vi "_Write.vi"(8 "error in (no error)":errorcluster, 9 "Timeout S (0)":dbl, 10 "Data":string, 11 "DeploySerialResource in":refnum<class "SerialResource.lvclass">) -> (0 "error out":errorcluster, 2 "Bytes Written":i32, 3 "DeploySerialResource out":refnum<class "SerialResource.lvclass">)   [LabVIEW 2020, in "PicoG-Core.lvlib" / "SerialResource.lvclass"]
uses:
  SerialResource.lvclass
  <vilib>/IlluminatedG/IG Serial Stream/Stream-Serial/Serial Client/Serial Client.lvclass
  <vilib>/IlluminatedG/lv-stream/stream/Stream.lvclass
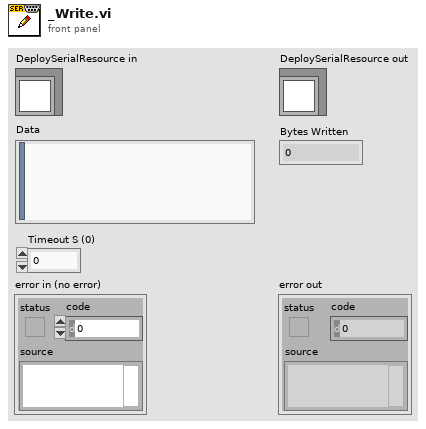
[diagram p1: front panel]
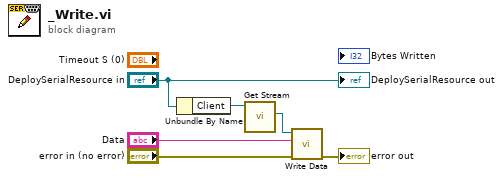
[diagram p0: block diagram]
diagram:
  n1 = Unbundle By Name("DeploySerialResource in") -> ("Client"=w5:refnum<class "Serial Client.lvclass">)
  n2 = call-dynamic "Get Stream.vi"("VISA Client in"=w5) -> ("Stream"=w4:refnum<class "Stream.lvclass">)  [unwired: 8 in, 2 out]
  n3 = call <vilib>:"Write Data.vi"("error in (no error)"="error in (no error)", "Data"="Data", "Stream in"=w4) -> ("error out"=→"error out":errorcluster)  [unwired: 7 in, 1 out]
  "DeploySerialResource out" <- "DeploySerialResource in"
